vi "mav_send_all.vi"(6 "flight mode":cluster{"f_mode":u16, "send":bool} {"f_mode" items=["MANUAL", "CIRCLE", "STABlLlZE", "TRAINING", "ACRO", "FBWA", "FBWB", "CRUISE", "AUTOTUNE", "-", "AUTO", "RTL", "LOITER", "TAKEOFF", "ADSB", "GUIDED", "-", "QSTABILIZE", "QHOVER", "QLOITER", "QLAND", "QRTL", "QAUTOTUNE", "QACRO", "THERMAL", "L TO QLAND"]}, 7 "arm disarm":cluster{"arm_disarm":u16, "send":bool} {"arm_disarm" items=["Force Arm", "Force Disarm", "Arm", "Disarm"]}, 8 "error in":errorcluster, 9 "Connection Type":enum32{"TCP", "SERIAL", "UDP"}(tab), 10 "packet_sequence_in":u8, 11 "mav_connection_in":T2) -> (0 "error out":errorcluster, 2 "packet_sequence_out":u8, 3 "mav_connection_out":T2)   [LabVIEW 2023]
panel:
  in  "STATUSTEXT":T1={"severity"=enum."MAV_SEVERITY_INFO", "id"=0, "chunk_seq"=0, "text"="Labview Ground Control Station 0.1", "self"={"system_id"=255, "component_id"=190}}
  in  "AUTOPILOT_VERSION_REQUEST":T3={"self"={"system_id"=255, "component_id"=190}, "target_system"=1, "target_component"=1}
  in  "timer_5000":u32
  in  "HEARTBEAT":T4={"self"={"system_id"=255, "component_id"=190}, "custom_mode"=0, "type"=enum."MAV_TYPE_GCS", "autopilot"=enum."MAV_AUTOPILOT_INVALID", "base_mode"=0, "system_status"=enum."MAV_STATE_UNINIT"}
  out "timer":u32
  in  "timer_1000":u32
  in  "REQUEST_DATA_STREAM":T5={"self"={"system_id"=255, "component_id"=190}, "target_system"=1, "target_component"=1, "req_stream_id"=0, "req_message_rate (Hz)"=30, "start_stop"=1}
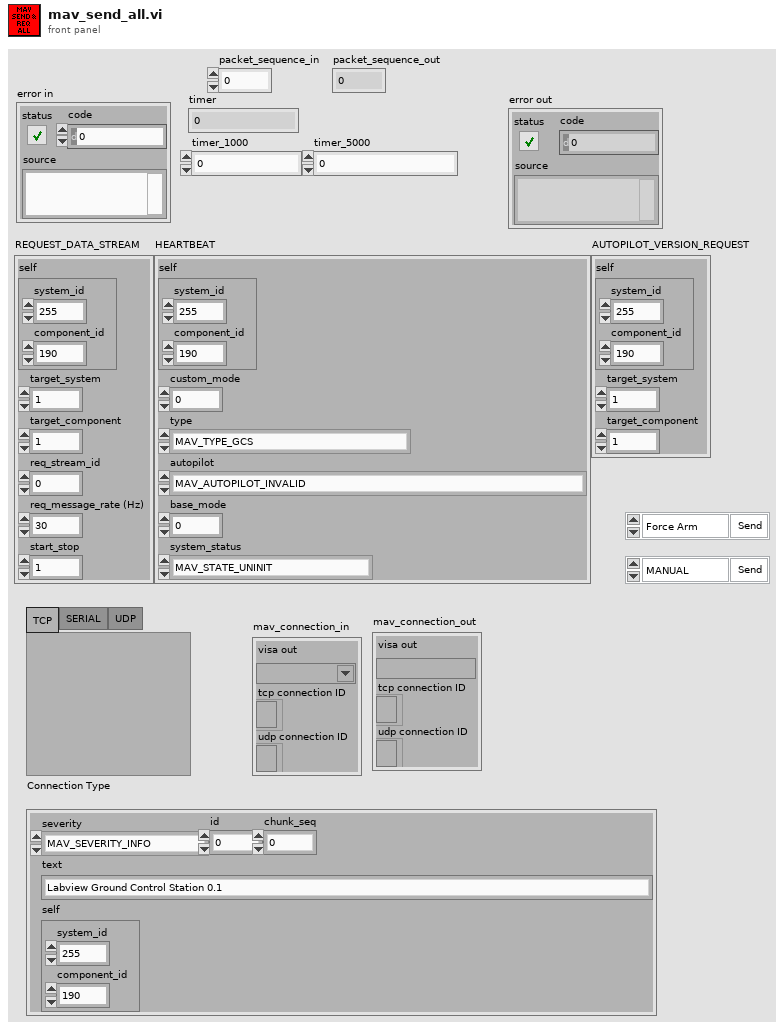
[diagram p1: front panel]
types:
  T1 = cluster{"severity":enum8{"MAV_SEVERITY_EMERGENCY", "MAV_SEVERITY_ALERT", "MAV_SEVERITY_CRITICAL", "MAV_SEVERITY_ERROR", "MAV_SEVERITY_WARNING", "MAV_SEVERITY_NOTICE", "MAV_SEVERITY_INFO", "MAV_SEVERITY_DEBUG"}, "id":u16, "chunk_seq":u8, "text":string, "self":cluster{"system_id":u8, "component_id":u8}}
  T2 = cluster{"visa out":refnum<visa-resource-name>, "tcp connection ID":refnum<k5>, "udp connection ID":refnum<k16>}
  T3 = cluster{"self":cluster{"system_id":u8, "component_id":u8}, "target_system":u8, "target_component":u8}
  T4 = cluster{"self":cluster{"system_id":u8, "component_id":u8}, "custom_mode":u32, "type":enum8{"MAV_TYPE_GENERIC", "MAV_TYPE_FIXED_WING", "MAV_TYPE_QUADROTOR", "MAV_TYPE_COAXIAL", "MAV_TYPE_HELICOPTER", "MAV_TYPE_ANTENNA_TRACKER", "MAV_TYPE_GCS", "MAV_TYPE_AIRSHIP", "MAV_TYPE_FREE_BALLOON", "MAV_TYPE_ROCKET", "MAV_TYPE_GROUND_ROVER", "MAV_TYPE_SURFACE_BOAT", "MAV_TYPE_SUBMARINE", "MAV_TYPE_HEXAROTOR", "MAV_TYPE_OCTOROTOR", "MAV_TYPE_TRICOPTER", "MAV_TYPE_FLAPPING_WING", "MAV_TYPE_KITE", "MAV_TYPE_ONBOARD_CONTROLLER", "MAV_TYPE_VTOL_TAILSITTER_DUOROTOR", "MAV_TYPE_VTOL_TAILSITTER_QUADROTOR", "MAV_TYPE_VTOL_TILTROTOR", "MAV_TYPE_VTOL_FIXEDROTOR", "MAV_TYPE_VTOL_TAILSITTER", "MAV_TYPE_VTOL_TILTWING", "MAV_TYPE_VTOL_RESERVED5", "MAV_TYPE_GIMBAL", "MAV_TYPE_ADSB", "MAV_TYPE_PARAFOIL", "MAV_TYPE_DODECAROTOR", "MAV_TYPE_CAMERA", "MAV_TYPE_CHARGING_STATION", "MAV_TYPE_FLARM", "MAV_TYPE_SERVO", "MAV_TYPE_ODID", "MAV_TYPE_DECAROTOR", "MAV_TYPE_BATTERY", "MAV_TYPE_PARACHUTE", "MAV_TYPE_LOG", "MAV_TYPE_OSD", "MAV_TYPE_IMU", "MAV_TYPE_GPS", "MAV_TYPE_WINCH", "MAV_TYPE_GENERIC_MULTIROTOR", "MAV_TYPE_ILLUMINATOR"}, "autopilot":enum8{"MAV_AUTOPILOT_GENERIC", "MAV_AUTOPILOT_RESERVED", "MAV_AUTOPILOT_SLUGS", "MAV_AUTOPILOT_ARDUPILOTMEGA", "MAV_AUTOPILOT_OPENPILOT", "MAV_AUTOPILOT_GENERIC_WAYPOINTS_ONLY", "MAV_AUTOPILOT_GENERIC_WAYPOINTS_AND_SIMPLE_NAVIGATION_ONLY", "MAV_AUTOPILOT_GENERIC_MISSION_FULL", "MAV_AUTOPILOT_INVALID", "MAV_AUTOPILOT_PPZ", "MAV_AUTOPILOT_UDB", "MAV_AUTOPILOT_FP", "MAV_AUTOPILOT_PX4", "MAV_AUTOPILOT_SMACCMPILOT", "MAV_AUTOPILOT_AUTOQUAD", "MAV_AUTOPILOT_ARMAZILA", "MAV_AUTOPILOT_AEROB", "MAV_AUTOPILOT_ASLUAV", "MAV_AUTOPILOT_SMARTAP", "MAV_AUTOPILOT_AIRRAILS", "MAV_AUTOPILOT_REFLEX"}, "base_mode":u8, "system_status":enum16{"MAV_STATE_UNINIT", "MAV_STATE_BOOT", "MAV_STATE_CALIBRATING", "MAV_STATE_STANDBY", "MAV_STATE_ACTIVE", "MAV_STATE_CRITICAL", "MAV_STATE_EMERGENCY", "MAV_STATE_POWEROFF", "MAV_STATE_FLIGHT_TERMINATION"}}
  T5 = cluster{"self":cluster{"system_id":u8, "component_id":u8}, "target_system":u8, "target_component":u8, "req_stream_id":u8, "req_message_rate (Hz)":u16, "start_stop":u8}
  T6 = cluster{"VISA out":refnum<visa-resource-name>, "tcp connection ID":refnum<k5>, "udp connection ID":refnum<k16>}
  T7 = cluster{"self":cluster{"system_id":u8, "component_id":u8}, "target_system":u8, "target_component":u8, "command (MAV_CMD)":u16, "confirmation":u8, "param1":sgl, "param2":sgl, "param3":sgl, "param4":sgl, "param5":sgl, "param6":sgl, "param7":sgl}
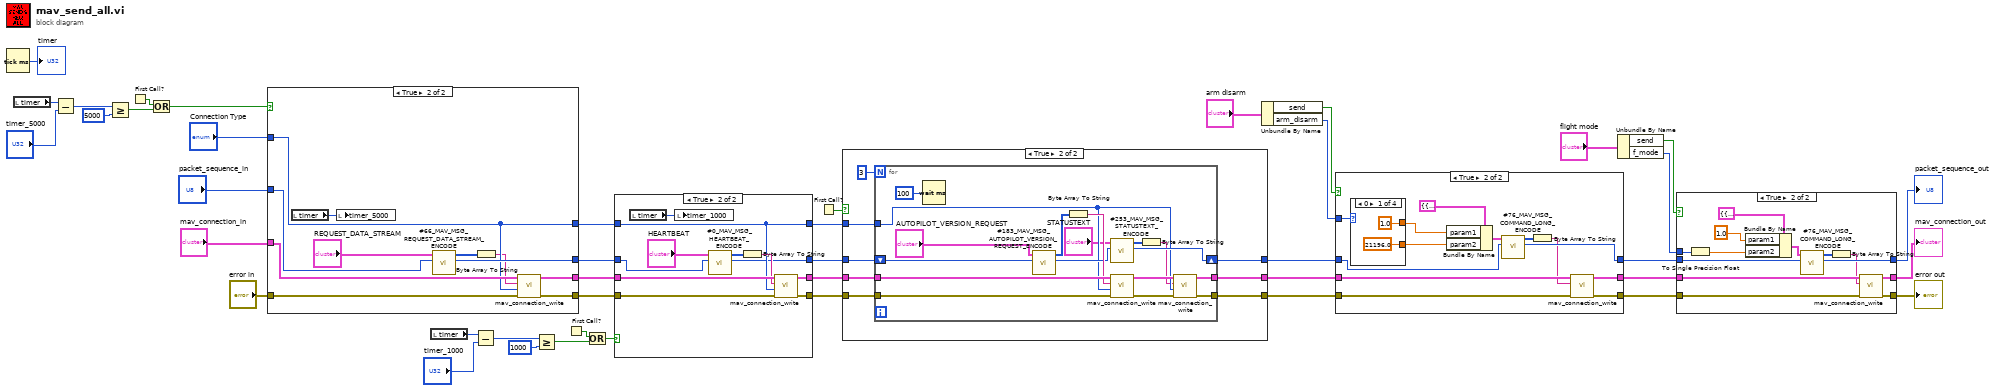
[diagram p0: block diagram]
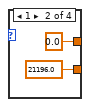
[diagram p4: hidden frame]
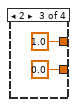
[diagram p5: hidden frame]
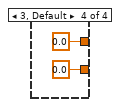
[diagram p6: hidden frame]
diagram:
  n1 = Tick Count (ms)() -> (millisecond timer value=→"timer":u32)
  n2 = local read "timer"() -> (w29:u32)
  n3 = Subtract(x=w29, y="timer_5000") -> (x-y=w32:u32)
  n4 = Greater Or Equal?(x=w32, y=u32 5000) -> (x >= y?=w30:bool)
  n5 = First Call?() -> (First Call?: T/F=w34:bool)
  n6 = Or(x=w34, y=w30) -> (x .or. y?=w33:bool)
  n7 = case shown="True" w33 {
    tunnel: "Connection Type" -> [w45 w52]
    tunnel: "error in" -> [w46 w58]
    tunnel: "mav_connection_in" -> [w47 w57]
    tunnel: "packet_sequence_in" -> [w44 w56]
    tunnel: [w47 w55] -> w36
    tunnel: [w46 w54] -> w35
    tunnel: [w44 w53] -> w38
    tunnel: [w45 w52] -> w37
    frame False {
    }
    frame True {
      n8 = local read "timer"() -> (w49:u32)
      n9 = local write "timer_5000"(w49) -> ()
      n10 = call "#66_MAV_MSG_REQUEST_DATA_STREAM_ENCODE.vi"("packet_sequence_in"=w56, "REQUEST_DATA_STREAM"="REQUEST_DATA_STREAM") -> ("packet_sequence_out"=w53:u8, "mavlink_buffer_out"=w48:u8[])  [unwired: 8 in]
      n11 = Byte Array To String(unsigned byte array=w48) -> (string=w51:string)
      n12 = call "mav_connection_write.vi"("error in"=w58, "Connection Type"=w52, "data in"=w51, "mav_connection_in"=w57) -> ("error out"=w54:errorcluster, "mav_connection_out"=w55:T6)  [unwired: 6 in]
    }
  }
  n13 = local read "timer"() -> (w26:u32)
  n14 = Subtract(x=w26, y="timer_1000") -> (x-y=w41:u32)
  n15 = Greater Or Equal?(x=w41, y=u32 1000) -> (x >= y?=w20:bool)
  n16 = First Call?() -> (First Call?: T/F=w21:bool)
  n17 = Or(x=w21, y=w20) -> (x .or. y?=w19:bool)
  n18 = case shown="True" w19 {
    tunnel: w37 -> [w62 w66]
    tunnel: [w60 w72] -> w23
    tunnel: [w61 w71] -> w24
    tunnel: w36 -> [w61 w70]
    tunnel: w35 -> [w60 w69]
    tunnel: [w62 w66] -> w16
    tunnel: w38 -> [w59 w65]
    tunnel: [w59 w64] -> w22
    frame False {
    }
    frame True {
      n19 = local read "timer"() -> (w73:u32)
      n20 = local write "timer_1000"(w73) -> ()
      n21 = call "#0_MAV_MSG_HEARTBEAT_ENCODE.vi"("packet_sequence_in"=w65, "HEARTBEAT"="HEARTBEAT") -> ("packet_sequence_out"=w64:u8, "mavlink_buffer_out"=w63:u8[])  [unwired: 8 in]
      n22 = Byte Array To String(unsigned byte array=w63) -> (string=w68:string)
      n23 = call "mav_connection_write.vi"("error in"=w69, "Connection Type"=w66, "data in"=w68, "mav_connection_in"=w70) -> ("error out"=w72:errorcluster, "mav_connection_out"=w71:T6)  [unwired: 6 in]
    }
  }
  n24 = First Call?() -> (First Call?: T/F=w25:bool)
  n25 = case shown="True" w25 {
    tunnel: w24 -> [w75 w84]
    tunnel: [w75 w83] -> w14
    tunnel: [w74 w82] -> w13
    tunnel: w23 -> [w74 w81]
    tunnel: w22 -> [w76 w80]
    tunnel: [w76 w79] -> w15
    tunnel: w16 -> [_ w77]
    frame False {
    }
    frame True {
      n26 = for {
        N: 3 -> [_]
        shift-right: [w93] -> w79
        shift-left: w80 -> [w97]
        tunnel: w84 -> [w101]
        tunnel: [w86] -> w83
        tunnel: w81 -> [w100]
        tunnel: [w85] -> w82
        tunnel: w77 -> [w89]
        n27 = Wait (ms)(milliseconds to wait=u32 100) -> ()  [unwired: 1 out]
        n28 = call "#183_MAV_MSG_AUTOPILOT_VERSION_REQUEST_ENCODE.vi"("packet_sequence_in"=w97, "AUTOPILOT_VERSION_REQUEST"="AUTOPILOT_VERSION_REQUEST") -> ("packet_sequence_out"=w94:u8, "mavlink_buffer_out"=w99:u8[])  [unwired: 8 in]
        n29 = Byte Array To String(unsigned byte array=w99) -> (string=w95:string)
        n30 = call "#253_MAV_MSG_STATUSTEXT_ENCODE.vi"("packet_sequence_in"=w94, "STATUSTEXT"="STATUSTEXT") -> ("packet_sequence_out"=w93:u8, "mavlink_buffer_out"=w92:u8[])  [unwired: 8 in]
        n31 = call "mav_connection_write.vi"("error in"=w100, "Connection Type"=w89, "data in"=w95, "mav_connection_in"=w101) -> ("error out"=w90:errorcluster, "mav_connection_out"=w91:T6)  [unwired: 6 in]
        n32 = Byte Array To String(unsigned byte array=w92) -> (string=w88:string)
        n33 = call "mav_connection_write.vi"("error in"=w90, "Connection Type"=w89, "data in"=w88, "mav_connection_in"=w91) -> ("error out"=w85:errorcluster, "mav_connection_out"=w86:T6)  [unwired: 6 in]
      }
    }
  }
  n34 = Unbundle By Name("arm disarm") -> ("send"=w11:bool, "arm_disarm"=w10:u16)
  n35 = case shown="True" w11 {
    tunnel: w15 -> [w104 w113]
    tunnel: [w104 w112] -> w2
    tunnel: [w102 w115] -> w4
    tunnel: [w103 w114] -> w7
    tunnel: w14 -> [w103 w117]
    tunnel: w13 -> [w102 w116]
    tunnel: w10 -> [_ w107]
    frame False {
    }
    frame True {
      n36 = case shown="0" w107 {
        tunnel: [sgl 1.0 ("param1") sgl 0.0 ("param1") sgl 1.0 ("param1") sgl 0.0 ("param1")] -> w106
        tunnel: [sgl 21196.0 ("param2") sgl 21196.0 ("param2") sgl 0.0 ("param2") sgl 0.0 ("param2")] -> w105
        frame 0 {
        }
        frame 1 {
        }
        frame 2 {
        }
        frame 3, Default {
        }
      }
      n37 = Bundle By Name(cluster=T7 {"self"={"system_id"=255, "component_id"=190}, "target_system"=1, "target_component"=1, "command (MAV_CMD)"=400, "confirmation"=0, "param1"=1.0, "param2"=0.0, "param3"=0.0, "param4"=0.0, "param5"=0.0, "param6"=0.0, "param7"=0.0} ("COMMAND_LONG"), "param1"=w106, "param2"=w105) -> (w108:T7)
      n38 = call "#76_MAV_MSG_COMMAND_LONG_ENCODE.vi"("packet_sequence_in"=w113, "COMMAND_LONG"=w108) -> ("packet_sequence_out"=w112:u8, "mavlink_buffer_out"=w111:u8[])  [unwired: 8 in]
      n39 = Byte Array To String(unsigned byte array=w111) -> (string=w110:string)
      n40 = call "mav_connection_write.vi"("error in"=w116, "data in"=w110, "mav_connection_in"=w117) -> ("error out"=w115:errorcluster, "mav_connection_out"=w114:T6)  [unwired: 7 in]
    }
  }
  n41 = Unbundle By Name("flight mode") -> ("send"=w8:bool, "f_mode"=w1:u16)
  n42 = case shown="True" w8 {
    tunnel: w2 -> [w128 w137]
    tunnel: [w128 w136] -> w3
    tunnel: [w126 w139] -> w5
    tunnel: [w127 w138] -> w6
    tunnel: w7 -> [w127 w141]
    tunnel: w4 -> [w126 w140]
    tunnel: w1 -> [_ w129]
    frame False {
    }
    frame True {
      n43 = To Single Precision Float(number=w129) -> (single precision float=w130:sgl)
      n44 = Bundle By Name(cluster=T7 {"self"={"system_id"=255, "component_id"=190}, "target_system"=1, "target_component"=1, "command (MAV_CMD)"=176, "confirmation"=0, "param1"=1.0, "param2"=0.0, "param3"=0.0, "param4"=0.0, "param5"=0.0, "param6"=0.0, "param7"=0.0} ("COMMAND_LONG"), "param1"=sgl 1.0, "param2"=w130) -> (w132:T7)
      n45 = call "#76_MAV_MSG_COMMAND_LONG_ENCODE.vi"("packet_sequence_in"=w137, "COMMAND_LONG"=w132) -> ("packet_sequence_out"=w136:u8, "mavlink_buffer_out"=w135:u8[])  [unwired: 8 in]
      n46 = Byte Array To String(unsigned byte array=w135) -> (string=w134:string)
      n47 = call "mav_connection_write.vi"("error in"=w140, "data in"=w134, "mav_connection_in"=w141) -> ("error out"=w139:errorcluster, "mav_connection_out"=w138:T6)  [unwired: 7 in]
    }
  }
  "error out" <- w5
  "packet_sequence_out" <- w3
  "mav_connection_out" <- w6
